vi "Start Main GUIs.vi"(8 "error in":errorcluster, 11 "cPAS Facade in":refnum<class "cPAS Facade.lvclass">) -> (0 "error out":errorcluster, 3 "cPAS Facade out":refnum<class "cPAS Facade.lvclass">)   [LabVIEW 2015, in "cPAS Facade.lvclass"]
uses:
  cPAS Facade.lvclass
  PAS/Class/PAS/Controls/PAS Control.lvclass
  PAS/Class/PAS/HF UI/PAS HF UI.lvclass
  PAS/Class/PAS/Derived/PAS Derived.lvclass
  CRDS/Controls/CRD Controls.lvclass
  CRDS/Ringdowns/CRD Ringdowns.lvclass
  CRDS/Derived Data/CRD Derived.lvclass
  Observer/cPAS Subject.lvclass
  PAS/Class/PAS/Housekeeping/PAS Housekeeping.lvclass
  CRDS/Housekeeping/CRD HK.lvclass
  Calibration/Calibration UI.lvclass
  CRDS/Data/cCRDS Data.lvclass
  Data/cPAS Data.lvclass
  Common/Common UI.lvclass
  Devices/CLAP/Data Subject/CLAP Subject.lvclass
  Pressure Calibration GUI/Pcal GUI.lvclass
  Observer/cCRD Subject/cCRD Subject.lvclass
  Reusable/GUI/Facade/GUI Facade.lvclass/GUI Facade.ctl
  Humidity Profile/Humidity Profile UI.lvclass
  Reusable/Observer/Observer.lvclass/Observer.ctl
  Reusable/GUI/GUI.lvclass/GUI.ctl
  Calibration/Calibration UI.lvclass/Calibration UI.ctl
  Reusable/Observer/Write Data Queue.vi
  Reusable/GUI/Accessors/Write Cmd Event.vi
  Calibration/Accessors/Write PAS DVR.vi
  Calibration/Accessors/Write CRD DVR.vi
  Reusable/GUI/Facade/Accessors/Write Data Subjects.vi
  Reusable/GUI/Facade/Accessors/Write GUIs.vi
  Reusable/GUI/Facade/Accessors/Write FP Refs.vi
  Reusable/Commands/Command.lvclass
  Reusable/Observer/Data Subject.lvclass
  Devices/CLAP/GUI/CLAP UI.lvclass
  Reusable/GUI/Facade/GUI Facade.lvclass
  Reusable/GUI/GUI.lvclass
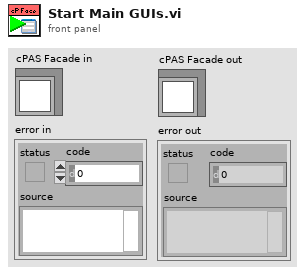
[diagram p1: front panel]
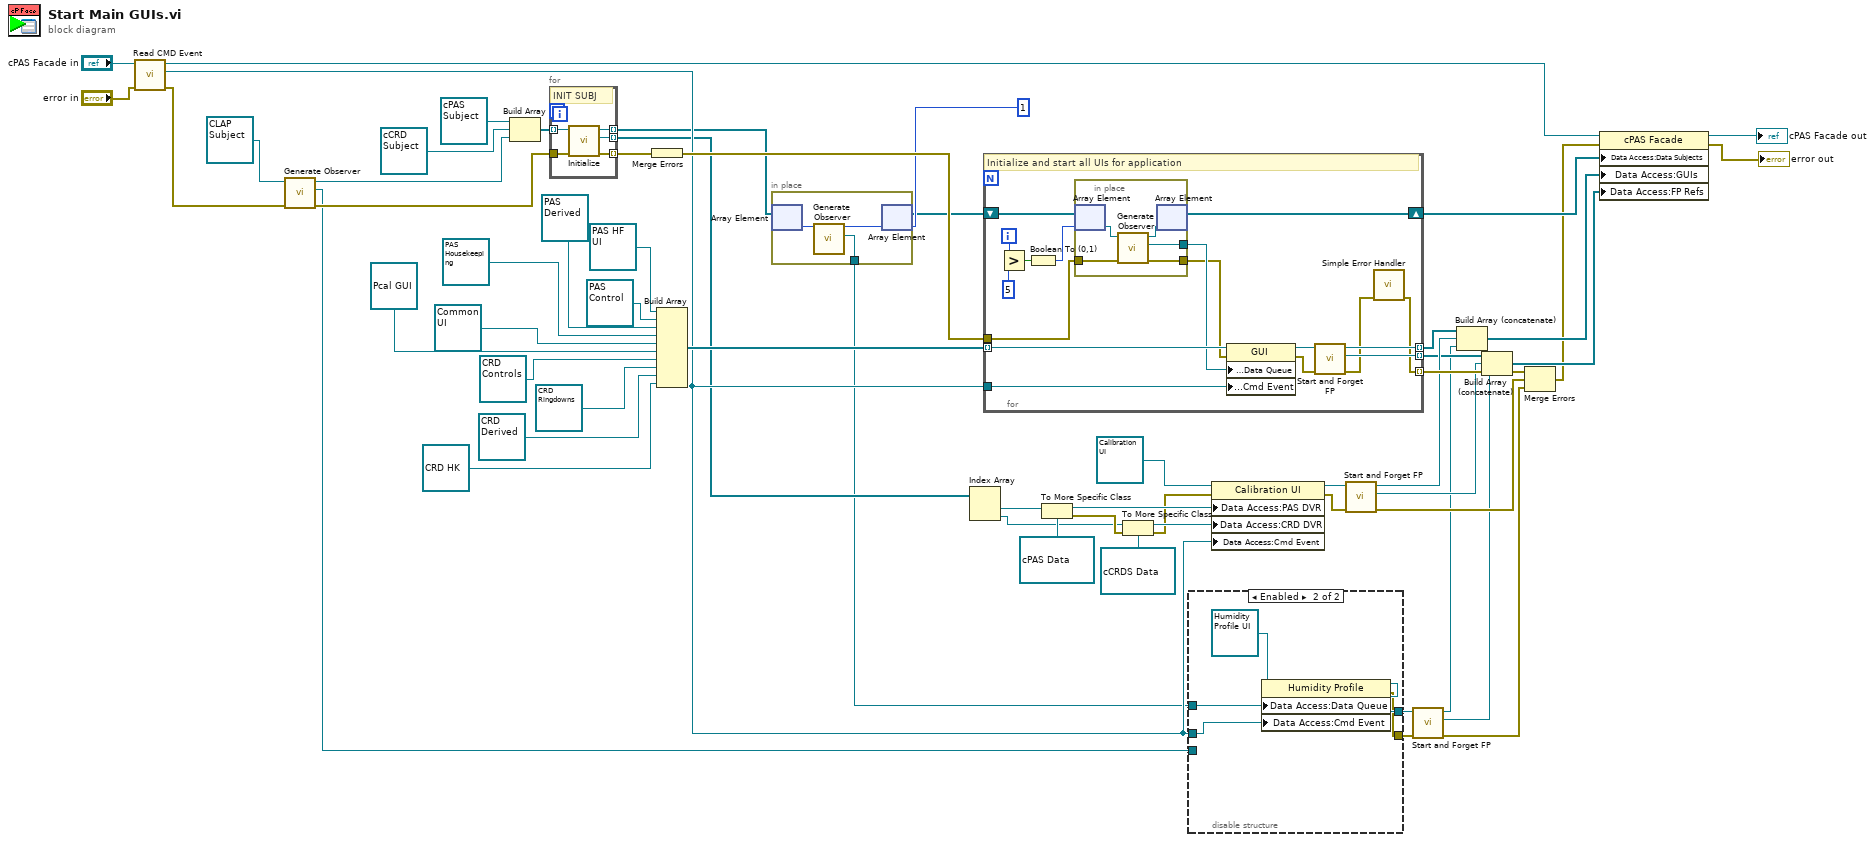
[diagram p0: block diagram]
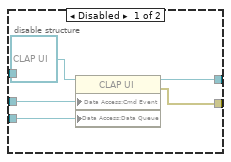
[diagram p2: hidden frame]
diagram:
  n1 = call "Read CMD Event.vi"("error in (no error)"="error in", "GUI Facade in"="cPAS Facade in") -> ("error out"=w13:errorcluster, "CMD Event"=w10:refnum<user-event>, "GUI Facade out"=w15:refnum<class "cPAS Facade.lvclass">)  [unwired: 7 in]
  n2 = call "Generate Observer.vi"("error in"=w13, "Data Subject in"=refnum<class "CLAP Subject.lvclass"> refnum ("CLAP Subject")) -> ("error out"=w22:errorcluster, "Observer"=w11:refnum<queue>, "Data Subject out"=w23:refnum<class "CLAP Subject.lvclass">)  [unwired: 7 in]
  n3 = Build Array(refnum<class "cPAS Subject.lvclass"> refnum ("cPAS Subj"), refnum<class "cCRD Subject.lvclass"> refnum ("cCRD Subject.lvclass"), w23) -> (w30:refnum<class "Data Subject.lvclass">[])
  n4 = for {
    tunnel: w30 -> [w63] mode=indexing
    tunnel: w22 -> [w62]
    tunnel: [w61] -> w3 mode=indexing
    tunnel: [w60] -> w5 mode=indexing
    tunnel: [w59] -> w28 mode=indexing
    # "INIT SUBJ"
    n5 = call-dynamic "Initialize.vi"("error in"=w62, "Data Subject in"=w63) -> ("error out"=w59:errorcluster, "DVR"=w60:refnum<data-value>, "Data Subject out"=w61:refnum<class "Data Subject.lvclass">)  [unwired: 7 in]
  }
  n6 = Merge Errors(w28) -> (w27:errorcluster)
  n7 = Build Array(refnum<class "PAS HF UI.lvclass"> refnum ("PAS HF UI"), refnum<class "PAS Control.lvclass"> refnum ("PAS Control"), refnum<class "PAS Derived.lvclass"> refnum ("PAS Derived.lvclass"), refnum<class "PAS Housekeeping.lvclass"> refnum ("PAS HK"), refnum<class "Common UI.lvclass"> refnum ("Common"), refnum<class "Pcal GUI.lvclass"> refnum ("Pcal GUI"), refnum<class "CRD Controls.lvclass"> refnum ("CRD Ctl UI"), refnum<class "CRD Ringdowns.lvclass"> refnum ("CRD Ringdowns.lvclass"), refnum<class "CRD Derived.lvclass"> refnum ("CRD Derived.lvclass"), refnum<class "CRD HK.lvclass"> refnum ("CRD HK")) -> (w38:refnum<class "GUI.lvclass">[])
  n8 = in-place {
    in-place-border: [w64] -> w1
    n9 = in-place-array #1(w3, 1) -> (w66:refnum<class "Data Subject.lvclass">)
    n10 = call "Generate Observer.vi"("Data Subject in"=w66) -> ("Observer"=w64:refnum<queue>, "Data Subject out"=w65:refnum<class "Data Subject.lvclass">)  [unwired: 8 in, 1 out]
    n11 = in-place-array #1(w65) -> (w2:refnum<class "Data Subject.lvclass">[])  [unwired: 1 out]
  }
  n12 = Index Array(array=w5) -> (element #1=w29:refnum<data-value>, element #2=w6:refnum<data-value>)  [unwired: 2 in]
  n13 = for {
    tunnel: w38 -> [w74] mode=indexing
    shift-right: [w82] -> w56
    shift-left: w2 -> [w83]
    tunnel: [w81] -> w43 mode=indexing
    tunnel: [w80] -> w46 mode=indexing
    tunnel: [w67] -> w57 mode=indexing
    tunnel: w27 -> [w79]
    tunnel: w10 -> [w69]
    i -> [w78]
    # "Initialize and start all UIs for application"
    n14 = Greater?(x=w78, y=5) -> (0:w76:bool)
    n15 = Boolean To (0,1)(Boolean=w76) -> (0, 1=w75:i16)
    n16 = in-place {
      in-place-border: [w86] -> w71
      in-place-border: [w85] -> w70
      in-place-border: w79 -> [w84]
      n17 = in-place-array #2(w83, w75) -> (w88:refnum<class "Data Subject.lvclass">)
      n18 = call "Generate Observer.vi"("error in"=w84, "Data Subject in"=w88) -> ("error out"=w85:errorcluster, "Observer"=w86:refnum<queue>, "Data Subject out"=w87:refnum<class "Data Subject.lvclass">)  [unwired: 7 in]
      n19 = in-place-array #2(w87) -> (w82:refnum<class "Data Subject.lvclass">[])  [unwired: 1 out]
    }
    n20 = property class="GUI"(reference=w74, error in=w70, "Data Access:Data Queue"=w71, "Data Access:Cmd Event"=w69) -> (reference out=w73:refnum<class "GUI.lvclass">, error out=w72:errorcluster)
    n21 = call "Start and Forget FP.vi"("error in"=w72, "GUI in"=w73) -> ("error out"=w68:errorcluster, "UI Ref"=w81:refnum<vi>, "GUI out"=w80:refnum<class "GUI.lvclass">)  [unwired: 6 in, 1 out]
    n22 = call <vilib>:"Simple Error Handler.vi"("error in (no error)"=w68) -> ("error out"=w67:errorcluster)  [unwired: 4 in, 4 out]
  }
  n23 = To More Specific Class(target class=refnum<data-value> refnum, reference=w29) -> (specific class reference=w49:refnum<data-value>, error out=w40:errorcluster)  [unwired: 1 in]
  n24 = To More Specific Class(target class=refnum<data-value> refnum, reference=w6, error in=w40) -> (specific class reference=w48:refnum<data-value>, error out=w39:errorcluster)
  n25 = disable-structure shown="Enabled" {
    disable-tunnel: [w92 w95] -> w12
    disable-tunnel: w11 -> [w91 _]
    disable-tunnel: w10 -> [w90 w96]
    disable-tunnel: [w89 w94] -> w9
    disable-tunnel: w1 -> [_ w97]
    frame Disabled {
      n26 = property class="CLAP UI"(reference=refnum<class "CLAP UI.lvclass"> refnum ("CLAP UI"), "Data Access:Cmd Event"=w90, "Data Access:Data Queue"=w91) -> (reference out=w92:refnum<class "CLAP UI.lvclass">, error out=w89:errorcluster)  [unwired: 1 in]
    }
    frame Enabled {
      n27 = property class="Humidity Profile"(reference=refnum<class "Humidity Profile UI.lvclass"> refnum ("Humidity Profile"), "Data Access:Data Queue"=w97, "Data Access:Cmd Event"=w96) -> (reference out=w95:refnum<class "Humidity Profile UI.lvclass">, error out=w94:errorcluster)  [unwired: 1 in]
    }
  }
  n28 = property class="Calibration UI"(reference=refnum<class "Calibration UI.lvclass"> refnum ("Calibration UI"), error in=w39, "Data Access:PAS DVR"=w49, "Data Access:CRD DVR"=w48, "Data Access:Cmd Event"=w10) -> (reference out=w51:refnum<class "Calibration UI.lvclass">, error out=w50:errorcluster)
  n29 = call "Start and Forget FP.vi"("error in"=w50, "GUI in"=w51) -> ("error out"=w47:errorcluster, "UI Ref"=w41:refnum<vi>, "GUI out"=w45:refnum<class "Calibration UI.lvclass">)  [unwired: 6 in, 1 out]
  n30 = call "Start and Forget FP.vi"("error in"=w9, "GUI in"=w12) -> ("error out"=w37:errorcluster, "UI Ref"=w36:refnum<vi>, "GUI out"=w35:refnum<class "Humidity Profile UI.lvclass">)  [unwired: 6 in, 1 out]
  n31 = Build Array (concatenate)(w46, w45, w35) -> (w44:refnum<class "GUI.lvclass">[])
  n32 = Build Array (concatenate)(w43, w41, w36) -> (w42:refnum<vi>[])
  n33 = Merge Errors(w57, w47, w37) -> (w7:errorcluster)
  n34 = property class="cPAS Facade"(reference=w15, error in=w7, "Data Access:Data Subjects"=w56, "Data Access:GUIs"=w44, "Data Access:FP Refs"=w42) -> (reference out=→"cPAS Facade out":refnum<class "cPAS Facade.lvclass">, error out=→"error out":errorcluster)
